vi "P2018 TB INCAR_Shutdown.vi"(8 "error in (no error)":errorcluster, 9 "Comunicaciones":T1={"Flujo_1"="ASRL6::INSTR", "Brk1"=FALSE, "Flujo_2"="ASRL6::INSTR", "Brk2"=FALSE, "Flujo_3"="ASRL6::INSTR", "Brk3"=FALSE, "Flujo_4"="ASRL6::INSTR", "Brk4"=FALSE, "Eurothe"="ASRL6::INSTR", "Eurot"=FALSE, "Balanza"="ASRL6::INSTR", "Bal"=FALSE, "eValPos"="ASRL6::INSTR", "eVal"=FALSE, "flowbus"="ASRL6::INSTR", "fb"=FALSE}) -> (0 "error out":errorcluster)   [LabVIEW 2013]
uses:
  Controles/P2018 Com Control.ctl
  serialTermobDisbal/Multicard III_Hardware_Module Control.ctl
  modbusEurotherm P116_485/Eurotherm_Hardware_Module Control.ctl
  serialArduinoMicro/ArduinoMicro Module Control.ctl
panel:
  # "Input"
  # "Output"
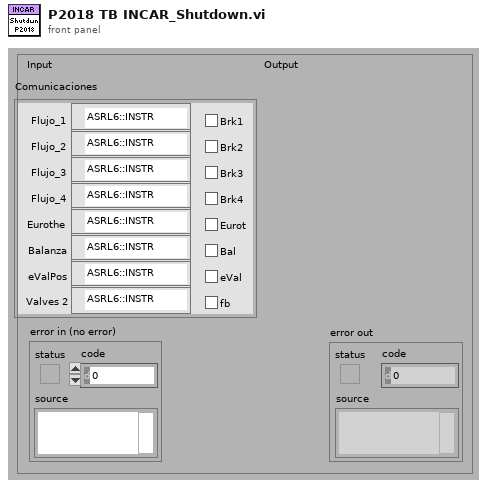
[diagram p1: front panel]
types:
  T1 = typedef "P2018 Com Control.ctl" = cluster{"Flujo_1":refnum<visa-resource-name>, "Brk1":bool, "Flujo_2":refnum<visa-resource-name>, "Brk2":bool, "Flujo_3":refnum<visa-resource-name>, "Brk3":bool, "Flujo_4":refnum<visa-resource-name>, "Brk4":bool, "Eurothe":refnum<visa-resource-name>, "Eurot":bool, "Balanza":refnum<visa-resource-name>, "Bal":bool, "eValPos":refnum<visa-resource-name>, "eVal":bool, "flowbus":refnum<visa-resource-name>, "fb":bool}
  T2 = typedef "ArduinoMicro Module Control.ctl" = enum16{"Initialize", "Read Data", "Write Data", "Enable", "Disable", "Shutdown"}
  T3 = typedef "Eurotherm_Hardware_Module Control.ctl" = enum16{"Initialize", "Write SP", "Read SP+PV", "Write Rate", "Set P", "Set I", "Set D", "Shutdown"}
  T4 = typedef "Multicard III_Hardware_Module Control.ctl" = enum16{"Initialize", "Cero", "Span", "Read ugr", "Read mgr", "Read A/D", "Read T", "Number readings", "Thermocouple type", "Status", "Shutdown"}
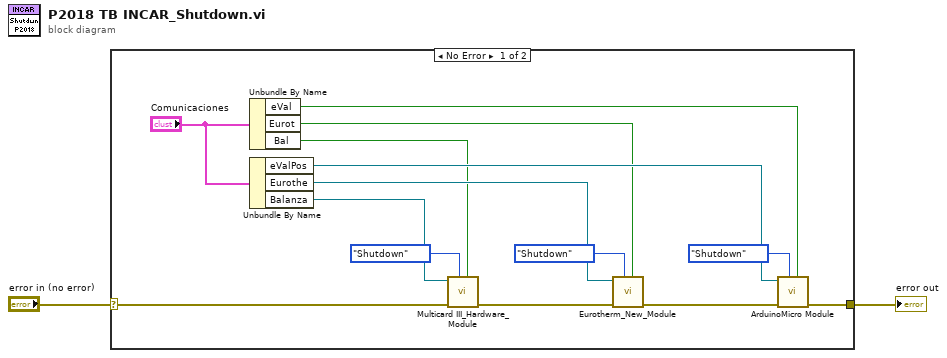
[diagram p0: block diagram]
diagram:
  n1 = case shown="No Error" "error in (no error)" {
    selector: "error in (no error)" -> [w10 w17]
    tunnel: [w8 w17] -> w1
    frame No Error {
      n2 = Unbundle By Name("Comunicaciones") -> ("eVal"=w3:bool, "Eurot"=w4:bool, "Bal"=w5:bool)
      n3 = Unbundle By Name("Comunicaciones") -> ("eValPos"=w6:refnum<visa-resource-name>, "Eurothe"=w11:refnum<visa-resource-name>, "Balanza"=w12:refnum<visa-resource-name>)
      n4 = call "Multicard III_Hardware_Module.vi"("Multicard (T:Enable)"=w5, "Command"=Multicard_III_Hardware_Module_Control."Shutdown", "error in (no error)"=w10, "VISA resource name"=w12) -> ("error out"=w13:errorcluster)  [unwired: 4 in, 3 out]
      n5 = call "Eurotherm_New_Module.vi"("Eurotherm (T:Enable)"=w4, "Command"=Eurotherm_Hardware_Module_Control."Shutdown", "error in (no error)"=w13, "VISA resource name"=w11) -> ("error out"=w9:errorcluster)  [unwired: 6 in, 1 out]
      n6 = call "ArduinoMicro Module.vi"("Enable"=w3, "Command"=ArduinoMicro_Module_Control."Shutdown", "error in (no error)"=w9, "VISA resource name"=w6) -> ("error out"=w8:errorcluster)  [unwired: 3 in, 4 out]
    }
    frame Error {
    }
  }
  "error out" <- w1
